vi "parse_header-single.vi"(8 "error in (no error)":errorcluster, 10 "header_to_get":string="Dropbox-Api-Result", 11 "headers":string) -> (0 "error out":errorcluster, 3 "value":string)   [LabVIEW 2015, in "lv-dropbox.lvlib"]
uses:
  lv-dropbox.lvlib
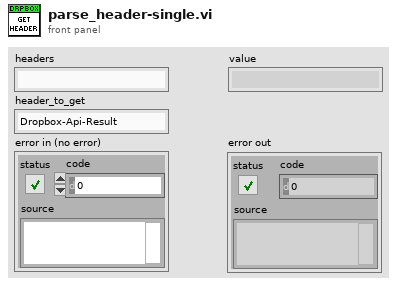
[diagram p1: front panel]
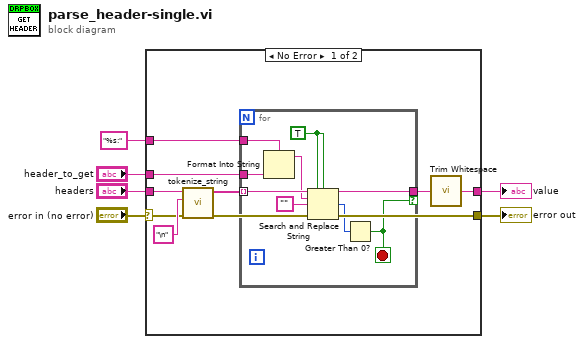
[diagram p0: block diagram]
diagram:
  n1 = case shown="No Error" "error in (no error)" {
    selector: "error in (no error)" -> [w13 w25]
    tunnel: [w11 w25] -> w2
    tunnel: "headers" -> [w15 _]
    tunnel: "header_to_get" -> [w10 _]
    tunnel: "%s:" -> [w9 _]
    tunnel: [w7 _] -> w1
    frame No Error {
      n2 = call "tokenize_string.vi"("error in (no error)"=w13, "delimiter"="\n", "input_string"=w15) -> ("error out"=w11:errorcluster, "delimited_string []"=w12:string[])  [unwired: 5 in, 2 out]
      n3 = for {
        tunnel: w12 -> [w22] mode=indexing
        tunnel: w10 -> [w23]
        tunnel: w9 -> [w24]
        tunnel: [w17] -> w8 if=w16
        stop <- w16 stop-if-true
        w21 = TRUE ("replace all? (F)")
        n4 = Format Into String(format string=w24, w23) -> (resulting string=w20:string)  [unwired: 2 in, 1 out]
        n5 = Search and Replace String(replace all?=w21, case sensitive?=w21, input string=w22, search string=w20, replace string="") -> (result string=w17:string, number of replacements=w18:i32)  [unwired: 3 in, 2 out]
        n6 = Greater Than 0?(x=w18) -> (x > 0?=w16:bool)
      }
      n7 = call <vilib>:"Trim Whitespace.vi"("string"=w8) -> ("trimmed string"=w7:string)  [unwired: 1 in]
    }
    frame Error {
    }
  }
  "error out" <- w2
  "value" <- w1
